vi "setSerializedData.vi"(0 "reference":refnum<class "ChoiceNode.lvclass">, 1 "parent":refnum<class "AbstractNode.lvclass">, 2 "children":refnum<class "AbstractNode.lvclass">[](array[class]), 3 "xmlOut":string, 5 "error in (no error)":errorcluster) -> (14 "reference out":refnum<class "ChoiceNode.lvclass">, 19 "error out":errorcluster)   [LabVIEW 2012, in "ChoiceNode.lvclass"]
doc: "setSerializedData"
uses:
  <resource>/Framework/Providers/Open_GDS/UML/ChoiceNode_class/ChoiceNode.lvclass
  <resource>/Framework/Providers/Open_GDS/UML/AbstractNode_class/AbstractNode.lvclass
  <resource>/Framework/Providers/Open_GDS/UML/AbstractNode_class/ObjectReference.ctl
  <resource>/Framework/Providers/Open_GDS/UML/General/Rectangle/Rectangle Rectangle2D.ctl
  <resource>/Framework/Providers/Open_GDS/UML/MultiLineString_class/ObjectReference.ctl
  <resource>/Framework/Providers/Open_GDS/UML/MultiLineString_class/MultiLineString.lvclass
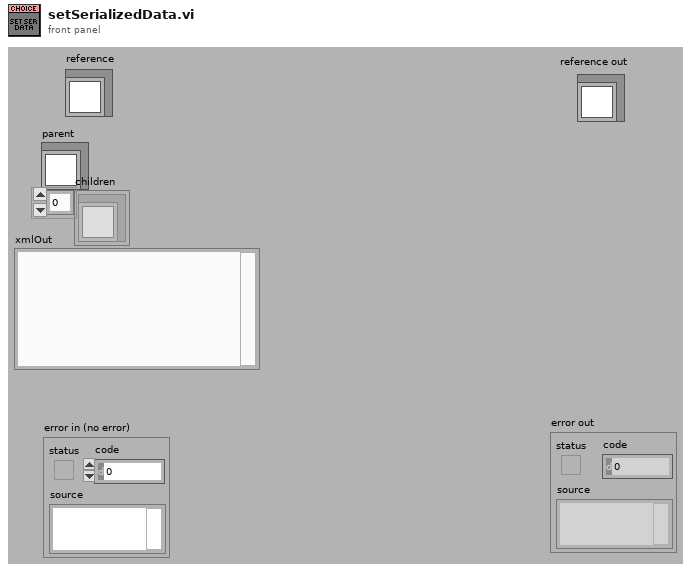
[diagram p1: front panel]
types:
  T1 = typedef "AbstractNode.lvclass/ObjectReference.ctl" = refnum<k1>
  T2 = typedef "Rectangle Rectangle2D.ctl" = cluster{"x":dbl, "y":dbl, "width":dbl, "height":dbl}
  T3 = typedef "MultiLineString.lvclass/ObjectReference.ctl" = refnum<k1>
  T4 = cluster{"Base class":cluster{"Base class":cluster{"parent":T1, "children":T1[]}, "bounds":T2}, "Text":T3, "DEFAULT_WIDTH":i32, "DEFAULT_HEIGHT":i32}
  T5 = typedef "ChoiceNode.lvclass/ObjectAttributes.ctl" = cluster{"Base class":T6, "Text":refnum<class "MultiLineString.lvclass">, "DEFAULT_WIDTH":i32, "DEFAULT_HEIGHT":i32}
  T6 = typedef "RectangularNode.lvclass/ObjectAttributes.ctl" = cluster{"Base class":T7, "bounds":T2}
  T7 = typedef "AbstractNode.lvclass/ObjectAttributes.ctl" = cluster{"parent":refnum<class "AbstractNode.lvclass">, "children":refnum<class "AbstractNode.lvclass">[], "Hidden":bool}
  T8 = cluster{"Attributes":cluster{"Base class":cluster{"Base class":cluster{"parent":T1, "children":T1[]}, "bounds":T2}, "Text":T3, "DEFAULT_WIDTH":i32, "DEFAULT_HEIGHT":i32}, string}
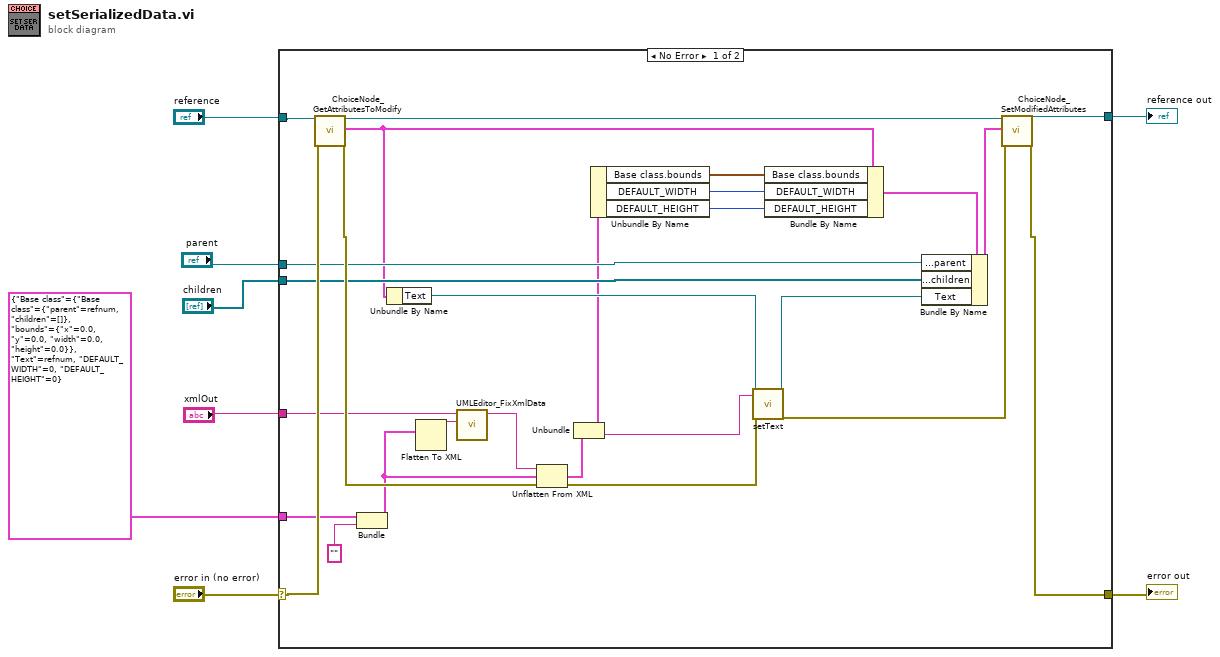
[diagram p0: block diagram]
diagram:
  n1 = case shown="No Error" "error in (no error)" {
    selector: "error in (no error)" -> [w26 w36]
    tunnel: "reference" -> [w27 w37]
    tunnel: [w25 w36] -> w6
    tunnel: [w24 w37] -> w5
    tunnel: "xmlOut" -> [w12 _]
    tunnel: "parent" -> [w23 _]
    tunnel: "children" -> [w22 _]
    tunnel: T4 {"Base class"={"Base class"={"parent"=refnum, "children"=[]}, "bounds"={"x"=0.0, "y"=0.0, "width"=0.0, "height"=0.0}}, "Text"=refnum, "DEFAULT_WIDTH"=0, "DEFAULT_HEIGHT"=0} ("Attributes") -> [w20 _]
    frame No Error {
      n2 = call <resource>:"ChoiceNode_GetAttributesToModify.vi"("reference in"=w27, "error in (no error)"=w26) -> ("reference out"=w35:refnum<class "ChoiceNode.lvclass">, "Attributes"=w14:T5, "error out"=w33:errorcluster)  [unwired: 1 in, 14 out]
      n3 = Bundle("Attributes"=w20, "") -> (w11:T8)  [unwired: 1 out]
      n4 = Unbundle By Name(w14) -> ("Text"=w32:refnum<class "MultiLineString.lvclass">)
      n5 = Flatten To XML(anything=w11) -> (xml string=w13:string)
      n6 = call <resource>:"UMLEditor_FixXmlData.vi"("XmlTemplateIn"=w13, "xmlIn"=w12) -> ("XML OUt"=w10:string)  [unwired: 9 in]
      n7 = Unflatten From XML(xml string=w10, type=w11, error in (no error)=w33) -> (value=w29:T8, error out=w31:errorcluster)
      n8 = Unbundle(w29) -> ("Attributes"=w16:T4, w28:string)
      n9 = Unbundle By Name(w16) -> ("Base class.bounds"=w19:T2, "DEFAULT_WIDTH"=w18:i32, "DEFAULT_HEIGHT"=w17:i32)
      n10 = call-dynamic "setText.vi"("reference"=w32, "text"=w28, "error in (no error)"=w31) -> ("reference out"=w30:refnum<class "MultiLineString.lvclass">, "error out"=w9:errorcluster)  [unwired: 15 out]
      n11 = Bundle By Name(cluster=w14, "Base class.bounds"=w19, "DEFAULT_WIDTH"=w18, "DEFAULT_HEIGHT"=w17) -> (w15:T5)
      n12 = Bundle By Name(cluster=w15, "Base class.Base class.parent"=w23, "Base class.Base class.children"=w22, "Text"=w30) -> (w34:T5)
      n13 = call <resource>:"ChoiceNode_SetModifiedAttributes.vi"("reference in"=w35, "Attributes"=w34, "error in (no error)"=w9) -> ("reference out"=w24:refnum<class "ChoiceNode.lvclass">, "error out"=w25:errorcluster)  [unwired: 3 in, 12 out]
    }
    frame Error {
    }
  }
  "reference out" <- w5
  "error out" <- w6
